vi "Get Variable Engine.vi"(8 "error in (no error)":errorcluster, 11 "App Properties in":refnum<class "App Properties.lvclass">) -> (0 "error out":errorcluster, 2 "Variable Engine":refnum<class "Variable Engine.lvclass">, 3 "App Properties out":refnum<class "App Properties.lvclass">)   [LabVIEW 2017]
uses:
  App Properties.lvclass
  C:/Program Files (x86)/National Instruments/LabVIEW 2017/vi.lib/TSS/ACRObat Test Framework/Classes/Base Objects/Base Class/Base Class/Class Properties/Class Properties.lvclass
  <vilib>/TSS/ACRObat Test Framework/Classes/Variable Engine/Class/Variable Engine.lvclass
  C:/Program Files (x86)/National Instruments/LabVIEW 2017/vi.lib/TSS/ACRObat Test Framework/Classes/Base Objects/Base Class/Base Class/Base Class.lvclass
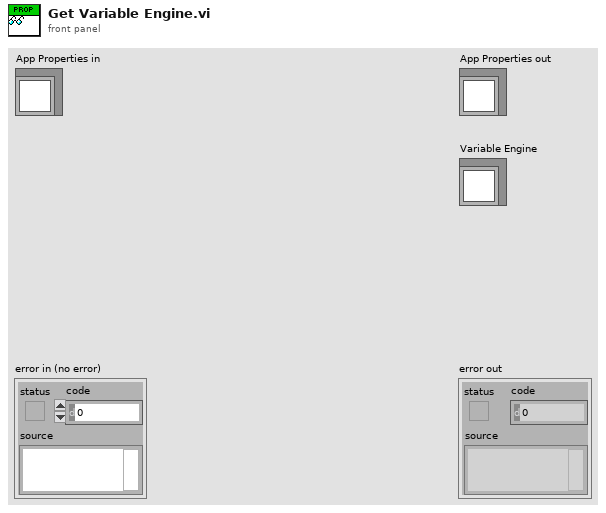
[diagram p1: front panel]
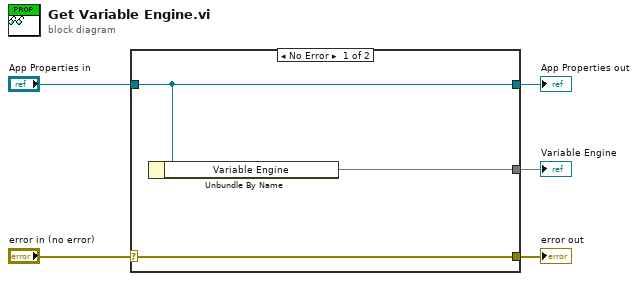
[diagram p0: block diagram]
diagram:
  n1 = case shown="No Error" "error in (no error)" {
    selector: "error in (no error)" -> [w8 w9]
    tunnel: [w8 w9] -> w4
    tunnel: [w7 w10] -> w2
    tunnel: "App Properties in" -> [w7 w10]
    tunnel: [w6 _] -> w1
    frame No Error {
      n2 = Unbundle By Name(w7) -> ("Variable Engine"=w6)
    }
    frame Error {
    }
  }
  "error out" <- w4
  "App Properties out" <- w2
  "Variable Engine" <- w1
